vi "CAN TDMS Writer.vi"   [LabVIEW 2015]
uses:
  Global Data.vi
types:
  T1 = enum16{"big-endian, network order", "native, host order", "little-endian"}
  T2 = enum16{"open", "open or create", "create or replace", "create", "open (read-only)"}
  T3 = cluster{"read mode":enum16{"polling", "blocking"}, "write mode":enum16{"polling", "blocking"}}
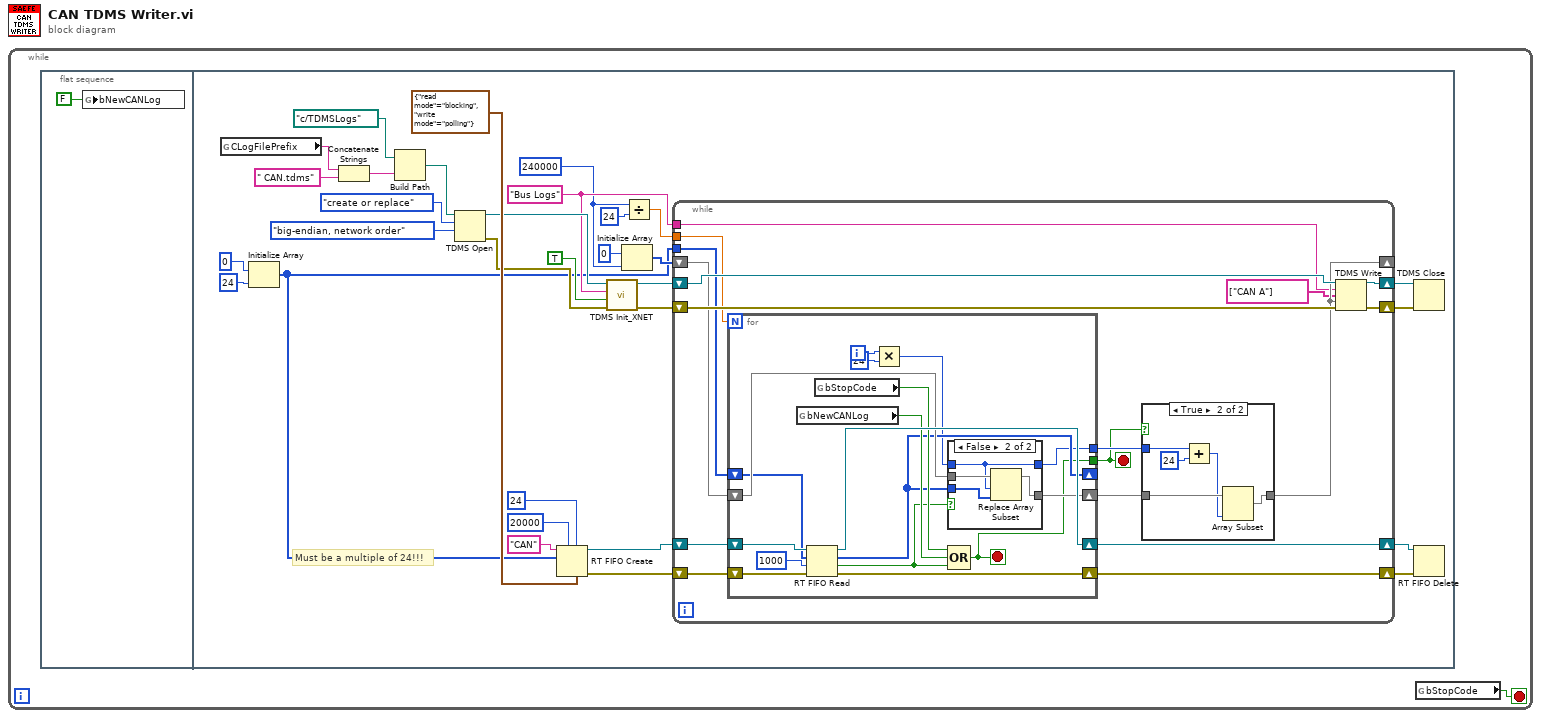
[diagram p0: block diagram]
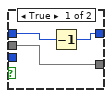
[diagram p3: hidden frame]
diagram:
  n1 = while {
    stop <- w1 stop-if-true
    n2 = flat-sequence {
      frame #0 {
        n3 = global write "Global Data.vi" "bNewCANLog"(FALSE ("New MC TDMS")) -> ()
      }
      frame #1 {
        w16 = "Bus Logs" ("group name")
        w5 = 240000 ("dimension size")
        # "Must be a multiple of 24!!!"
        n4 = global read "Global Data.vi" "CLogFilePrefix"() -> (w20:string)
        n5 = Initialize Array(u8 0 ("element"), 24 ("dimension size")) -> (w9:u8[])
        n6 = Concatenate Strings(w20, " CAN.tdms" ("string")) -> (w19:string)
        n7 = Build Path(base path=path "c:/TDMSLogs", name or relative path=w19) -> (appended path=w23:path)
        n8 = TDMS Open(9:T1."big-endian, network order" ("byte order (2:little-endian)"), 10:T2."create or replace" ("operation (0:open)"), 11:w23) -> (0:w15:errorcluster, 3:w17:refnum<k34>)  [unwired: 4 in]
        n9 = RT FIFO Create(0:"CAN" ("name (unnamed)"), 1:w9, 4:u32 20000 ("size (10)"), 6:u32 24 ("elements in array (1)"), 7:T3 {"read mode"=enum."blocking", "write mode"=enum."polling"} ("r/w modes (polling,polling)")) -> (8:w32:refnum<k33>, 11:w31:errorcluster)  [unwired: 3 in, 1 out]
        n10 = call "TDMS Init_XNET.vi"("error in (no error)"=w15, "sbRIO?"=TRUE, "group name"=w16, "tdms file"=w17) -> ("error out"=w14:errorcluster, "tdms file out"=w13:refnum<k34>)  [unwired: 6 in]
        n11 = Initialize Array(u8 0 ("element"), w5) -> (w28:u8[])
        n12 = Divide(x=w5, y=24) -> (x/y=w3:dbl)
        n13 = while {
          shift-right: [w42] -> _
          shift-left: w28 -> [w44]
          shift-right: [w48] -> w25
          shift-left: w32 -> [w50]
          shift-right: [w47] -> w24
          shift-left: w31 -> [w49]
          shift-right: [w39] -> w26
          shift-left: w13 -> [w46]
          shift-right: [w38] -> w27
          shift-left: w14 -> [w45]
          tunnel: w9 -> [w37]
          tunnel: w3 -> [w36]
          tunnel: w16 -> [w35]
          stop <- w34 stop-if-true
          n14 = for {
            N: w36 -> [_]
            shift-right: [w71] -> w48
            shift-left: w50 -> [w73]
            shift-right: [w70] -> w47
            shift-left: w49 -> [w72]
            shift-right: [w67] -> w43
            shift-left: w44 -> [w68]
            tunnel: [w57] -> w41
            shift-right: [w63] -> _
            shift-left: w37 -> [w64]
            tunnel: [w59] -> w34
            i -> [w62]
            stop <- w59 stop-if-true
            n15 = global read "Global Data.vi" "bNewCANLog"() -> (w65:bool)
            n16 = RT FIFO Read(0:w73, 1:w64, 2:1000 ("timeout in ms (0)"), 3:w72) -> (8:w71:refnum<k33>, 9:w63:u8[], 10:w58:bool, 11:w70:errorcluster)  [unwired: 1 out]
            n17 = global read "Global Data.vi" "bStopCode"() -> (w66:bool)
            n18 = Multiply(x=w62, y=24) -> (x*y=w61:i32)
            n19 = case shown="False" w58 {
              tunnel: w68 -> [w76 w80]
              tunnel: [w76 w79] -> w67
              tunnel: w63 -> [_ w78]
              tunnel: w61 -> [w75 w77]
              tunnel: [w74 w77] -> w57
              frame True {
                n20 = Decrement(x=w75) -> (x-1=w74:i32)
              }
              frame False {
                n21 = Replace Array Subset(array=w80, new element=w78, index=w77) -> (w79:u8[])
              }
            }
            n22 = Compound Arithmetic op=OR(w66, w65, w58) -> (w59:bool)
          }
          n23 = case shown="True" w34 {
            tunnel: w43 -> [w51 w56]
            tunnel: [w51 w55] -> w42
            tunnel: w41 -> [_ w54]
            frame False {
            }
            frame True {
              n24 = Add(x=w54, y=24) -> (x+y=w52:i32)
              n25 = Array Subset(array=w56, length=w52) -> (w55:u8[])  [unwired: 1 in]
            }
          }
          n26 = TDMS Write(0:w46, 5:w35, 7:string[] ["CAN A"], 9:w42, 11:w45) -> (4:w39:refnum<k34>, 15:w38:errorcluster)  [unwired: 1 in, 2 out]
        }
        n27 = TDMS Close(8:w27, 11:w26) -> ()  [unwired: 2 out]
        n28 = RT FIFO Delete(0:w25, 3:w24) -> ()  [unwired: 1 in, 1 out]
      }
    }
    n29 = global read "Global Data.vi" "bStopCode"() -> (w1:bool)
  }
